vi "dfd_Convert Wordlength to DataType.vi"(4 "Data wl":i16) -> (1 "Data Type":T1=-2 items=["U32"=4, "I32"=-4, "U16"=2, "I16"=-2, "U8"=1, "I8"=-1, "Boolean"=0, "Void"=10])   [LabVIEW 2017, in "NI_DigFilterLicensed.lvlib"]
uses:
  <vilib>/addons/Digital Filter Design/NI_DigFilterLicensed.lvlib
  <vilib>/rvi/ClientSDK/Core/Script/Fifo/ProjectItem/Public/nirviPiFifoType_DataTypes.ctl
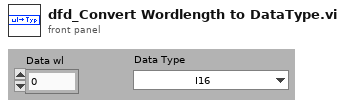
[diagram p1: front panel]
types:
  T1 = typedef "nirviPiFifoType_DataTypes.ctl" = i16
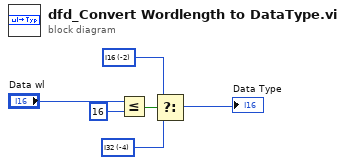
[diagram p0: block diagram]
diagram:
  w1 = T1 -4 items=["U32"=4, "I32"=-4, "U16"=2, "I16"=-2, "U8"=1, "I8"=-1, "Boolean"=0, "Void"=10] ("Data Type")
  w2 = T1 -2 items=["U32"=4, "I32"=-4, "U16"=2, "I16"=-2, "U8"=1, "I8"=-1, "Boolean"=0, "Void"=10] ("Data Type")
  n1 = Less Or Equal?(x="Data wl", y=i16 16) -> (x <= y?=w3:bool)
  n2 = Select(t=w2, s=w3, f=w1) -> (s? t:f=→"Data Type":T1)
